vi "Load-file.vi"(8 "error in (no error)":errorcluster, 11 "Object ref in":T1) -> (0 "error out":errorcluster, 3 "Object ref out":T1)   [LabVIEW 2013, in "HardwareCharacterization.lvlib" / "HC-Main.lvclass"]
uses:
  HC-Main.lvclass
  Object-reference.ctl
  Application-status.ctl
  UI/Control-names.ctl
  HC-Main.lvclass/HC-Main.ctl
  ScanParser/HC-ScanParser.lvclass/HC-ScanParser.ctl
  Read UI.vi
  Read Parser.vi
  Read Scan file path.vi
  ScanParser/Write Scan file path.vi
  UI/Set-control-enable-single.vi
  UI/HC-UI.lvclass
  ScanParser/HC-ScanParser.lvclass
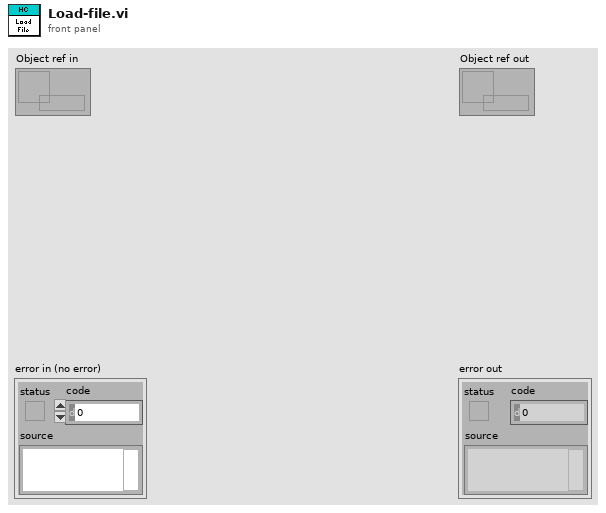
[diagram p1: front panel]
types:
  T1 = typedef "HardwareCharacterization.lvlib/HC-Main.lvclass/Object-reference.ctl" = refnum<data-value>
  T2 = typedef "HardwareCharacterization.lvlib/HC-UI.lvclass/Control-names.ctl" = enum16{"Help", "Status", "Load configuration", "Save configuration", "Activate", "Start", "Stop", "Options"}
  T3 = typedef "HardwareCharacterization.lvlib/HC-Main.lvclass/Application-status.ctl" = enum16{"Idle", "Initialized", "Configured", "Activated", "Started", "Paused", "Stopped", "Reset", "Error", "Exited"}
  T4 = typedef "HardwareCharacterization.lvlib/HC-UI.lvclass/Panes-reference.ctl" = refnum<data-value>
  T5 = typedef "HardwareCharacterization.lvlib/HC-ScanParser.lvclass/Object-reference.ctl" = refnum<data-value>
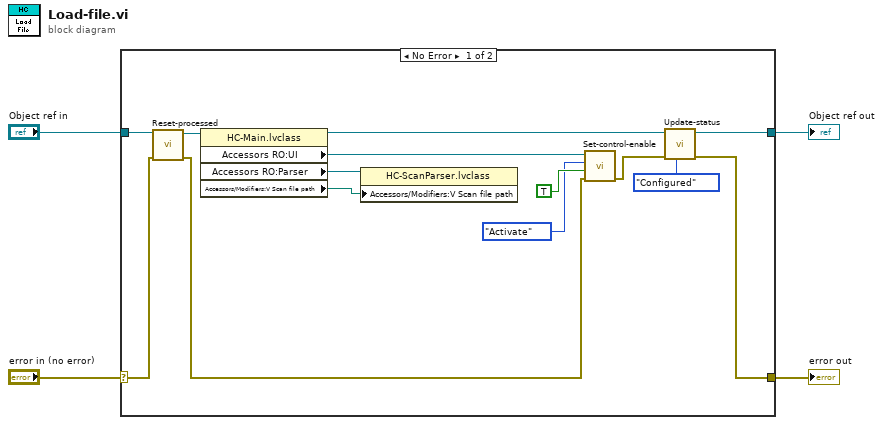
[diagram p0: block diagram]
diagram:
  n1 = case shown="No Error" "error in (no error)" {
    selector: "error in (no error)" -> [w10 w20]
    tunnel: [w5 w20] -> w3
    tunnel: [w8 w19] -> w1
    tunnel: "Object ref in" -> [w12 w19]
    frame No Error {
      n2 = call "Reset-processed.vi"("error in (no error)"=w10, "Object ref in"=w12) -> ("error out"=w6:errorcluster, "Object ref out"=w11:T1)  [unwired: 8 in]
      n3 = property class="HC-Main.lvclass"(reference=w11) -> (reference out=w9:T1, "Accessors RO:UI"=w7:T4, "Accessors RO:Parser"=w13:T5, "Accessors/Modifiers:V Scan file path"=w18:path)  [unwired: 1 in, 1 out]
      n4 = property class="HC-ScanParser.lvclass"(reference=w13, "Accessors/Modifiers:V Scan file path"=w18) -> ()  [unwired: 1 in, 2 out]
      n5 = call-poly "Set-control-enable.vi"("error in (no error)"=w6, "Enable?"=TRUE, "Control name"=Control-names."Activate", "Panes in"=w7) -> ("error out"=w14:errorcluster)  [unwired: 6 in, 1 out]
      n6 = call "Update-status.vi"("Status"=Application-status."Configured", "error in (no error)"=w14, "Object ref in"=w9) -> ("error out"=w5:errorcluster, "Object ref out"=w8:T1)  [unwired: 7 in]
    }
    frame Error {
    }
  }
  "error out" <- w3
  "Object ref out" <- w1
